vi "FGA COP Map Add Position.vi"(0 "LocalPose":T1) -> ()   [LabVIEW 2009]
uses:
  Support Files/LocalPose.ctl
  Support Files/TimeRec.ctl
  cRIO/Functional Global Variables/Actions for FG's.ctl
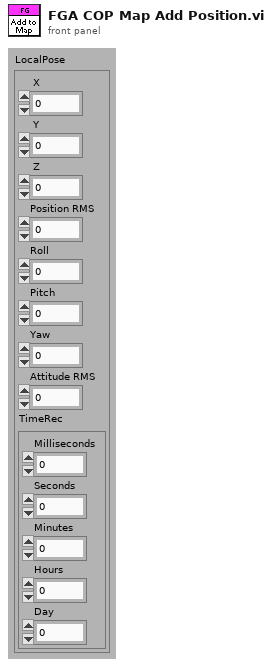
[diagram p1: front panel]
types:
  T1 = typedef "LocalPose.ctl" = cluster{" X":dbl, " Y":dbl, " Z":dbl, "Position RMS":dbl, "Roll":dbl, "Pitch":dbl, "Yaw":dbl, "Attitude RMS":dbl, "TimeRec":T2}
  T2 = typedef "TimeRec.ctl" = cluster{"Milliseconds":u32, "Seconds":u32, "Minutes":u32, "Hours":u32, "Day":u32}
  T3 = typedef "Actions for FG's.ctl" = enum16{"Read", "Write"}
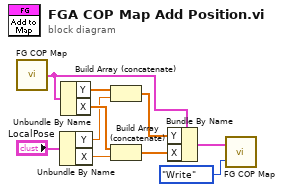
[diagram p0: block diagram]
diagram:
  n1 = call "FG COP Map.vi"() -> ("Map out"=w5:cluster{"Y":dbl[], "X":dbl[]})  [unwired: 2 in]
  n2 = Unbundle By Name("LocalPose") -> ("Y"=w7:dbl, "X"=w6:dbl)
  n3 = Unbundle By Name(w5) -> ("Y"=w10:dbl[], "X"=w9:dbl[])
  n4 = Build Array (concatenate)(w10, w7) -> (w4:dbl[])
  n5 = Build Array (concatenate)(w9, w6) -> (w3:dbl[])
  n6 = Bundle By Name(cluster=w5, "Y"=w4, "X"=w3) -> (w2:cluster{"Y":dbl[], "X":dbl[]})
  n7 = call "FG COP Map.vi"("FG Action (Read)"=Actions_for_FG's."Write", "Map in"=w2) -> ()  [unwired: 1 out]
